vi "WriteToConsole.vi"() -> ()   [LabVIEW 2020]
panel:
  in  "string":string
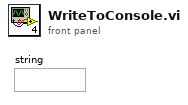
[diagram p1: front panel]
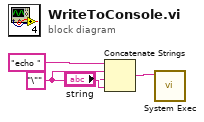
[diagram p0: block diagram]
diagram:
  w2 = "\"" ("string")
  n1 = Concatenate Strings("echo " ("string"), w2, "string", w2) -> (w3:string)
  n2 = call <vilib>:"System Exec.vi"("command line"=w3) -> ()  [unwired: 7 in, 4 out]
